vi "所有因子(I32).vi"(1 "范围":i32) -> (0 "所有因子":i32[](array[numeric]))   [LabVIEW 2012]
doc: "功能：\n\n求完数。\n\n完数的定义：\n\n一个数如果恰好等于它的因子之和，则这个数称作“完数”，比如：\n6=1+2+3\n\ncsxcs_366创建"
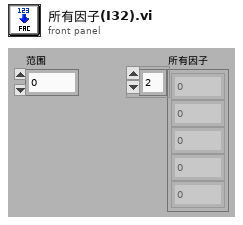
[diagram p1: front panel]
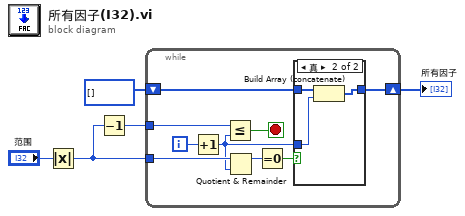
[diagram p0: block diagram]
diagram:
  n1 = Absolute Value(x="范围") -> (abs(x)=w2:i32)
  n2 = Decrement(x=w2) -> (x-1=w1:i32)
  n3 = while {
    tunnel: w2 -> [w12]
    shift-right: [w8] -> w3
    shift-left: i32[] [] -> [w9]
    tunnel: w1 -> [w6]
    i -> [w14]
    stop <- w13 stop-if-true
    n4 = Increment(x=w14) -> (x+1=w7:i32)
    n5 = Less Or Equal?(x=w6, y=w7) -> (x <= y?=w13:bool)
    n6 = Quotient & Remainder(x=w12, y=w7) -> (x-y*floor(x/y)=w11:i32)  [unwired: 1 out]
    n7 = Equal To 0?(x=w11) -> (x = 0?=w10:bool)
    n8 = case shown="真" w10 {
      tunnel: w9 -> [w15 w18]
      tunnel: [w15 w16] -> w8
      tunnel: w7 -> [_ w17]
      frame False {
      }
      frame True {
        n9 = Build Array (concatenate)(w18, w17) -> (w16:i32[])
      }
    }
  }
  "所有因子" <- w3
